vi "CSM - MassData Parameter Status.vi"(8 "Error in":errorcluster caption="Error in (no error)") -> (1 "Error out":errorcluster, 2 "Active Read Operation":T1, 3 "Active Write Operation":T1, 4 "Cache Size":i32)   [LabVIEW 2017, in "CSM MassData Parameter Support.lvlib"]
doc: "Reads the status information of the Massdata background cache.\n\n-- <b>Indicators</b> --\n- <b>Active Read Operation</b>: Information about the last read operation, including start address and length.\n- <b>Active Write Operation</b>: Information about the last write operation, including start address and length.\n- <b>Cache Size</b>: Background cache size in bytes."
uses:
  CSM MassData Parameter Support.lvlib
  _support/Def-MassDataOper-Status.ctl
  _support/Operation-FGV-MassData.ctl
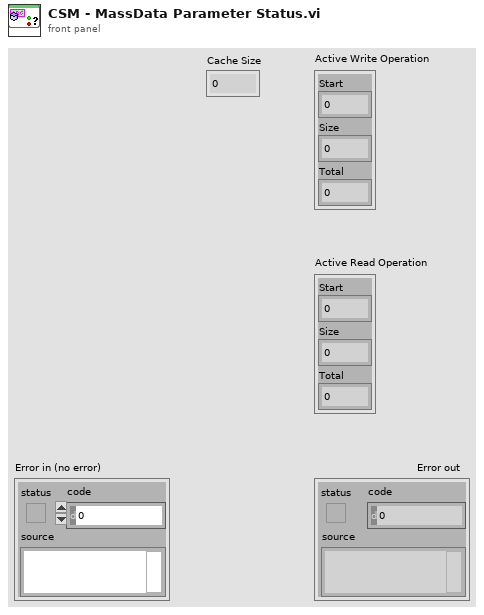
[diagram p1: front panel]
types:
  T1 = typedef "CSM MassData Parameter Support.lvlib/Def-MassDataOper-Status.ctl" = cluster{"Start":i32, "Size":i32, "Total":i32}
  T2 = typedef "CSM MassData Parameter Support.lvlib/Operation-FGV-MassData.ctl" = enum16{"Initialize", "Read", "Write", "Status", "Release"}
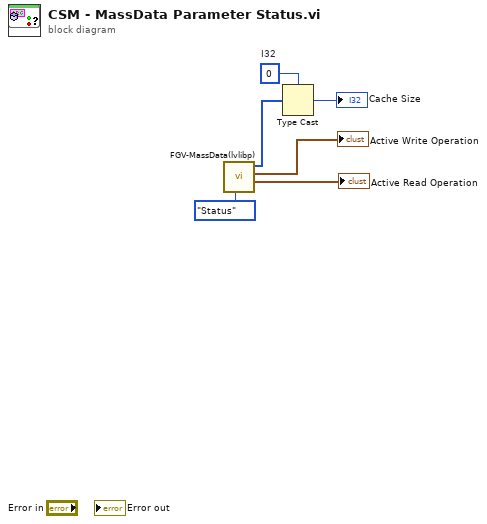
[diagram p0: block diagram]
diagram:
  w1 = 0  # I32
  n1 = call "FGV-MassData(lvlibp).vi"("Operation"=Operation-FGV-MassData."Status") -> ("Active Read Oper"=→"Active Read Operation":T1, "Active Write Oper"=→"Active Write Operation":T1, "Data out"=w3:u8[])  [unwired: 7 in, 1 out]
  n2 = Type Cast(type=w1, x=w3) -> (*(type *) &x=→"Cache Size":i32)
